vi "ParseErrorCore.vi"(8 "error in (no error)":errorcluster, 11 "LabErrorUX in":refnum<class "LabErrorUX.lvclass">) -> (0 "error out":errorcluster, 2 "ErrorUX":T1, 3 "LabErrorUX out":refnum<class "LabErrorUX.lvclass">)   [LabVIEW 2019, in "LabErrorUX.lvclass"]
uses:
  LabErrorUX.lvclass
  LabErrorUX.lvclass/LabErrorUX.ctl
  Typedefs/ErrorUX.ctl
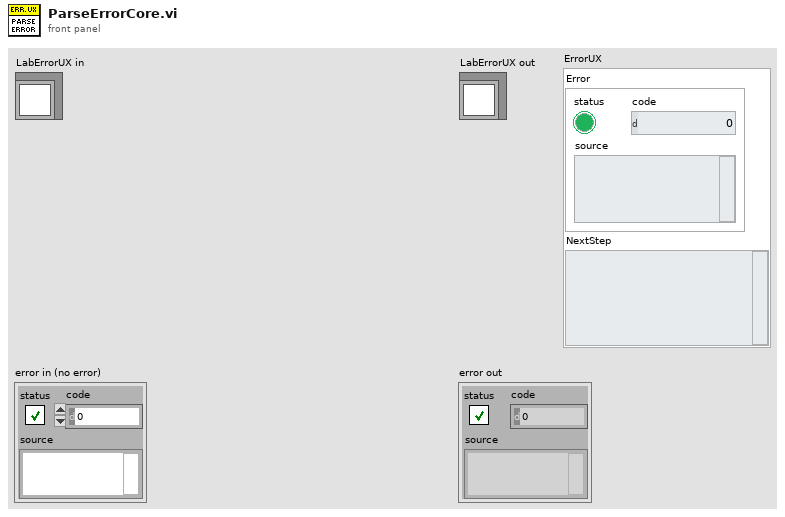
[diagram p1: front panel]
types:
  T1 = typedef "LabErrorUX.lvclass/ErrorUX.ctl" = cluster{"Error":errorcluster, "NextStep":string}
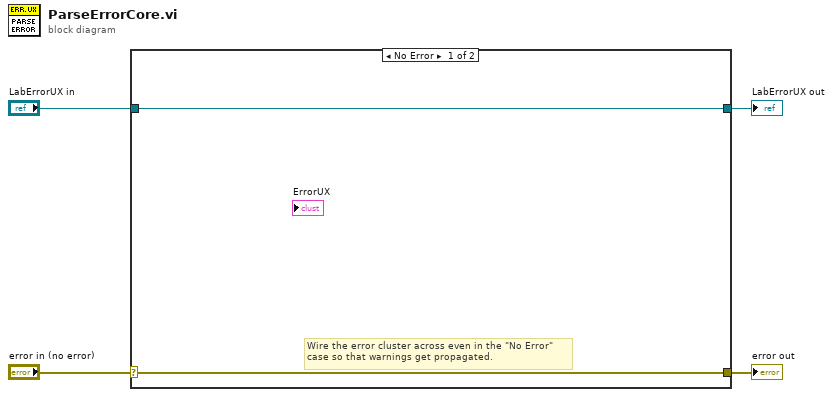
[diagram p0: block diagram]
diagram:
  n1 = case shown="No Error" "error in (no error)" {
    selector: "error in (no error)" -> [w5 w8]
    tunnel: [w5 w8] -> w3
    tunnel: [w6 w7] -> w1
    tunnel: "LabErrorUX in" -> [w6 w7]
    frame No Error {
      # "Wire the error cluster across even in the \"No Error\"\ncase so that warnings get propagated."
    }
    frame Error {
    }
  }
  "error out" <- w3
  "LabErrorUX out" <- w1
